vi "IT8800-Configure Range.vi"(6 "Numeric":dbl format="%#_13g", 8 "error in":errorcluster, 9 "Range":u16(ring) items=["MIN", "MAX", "DEFAULT"], 10 "Range Type":T2, 11 "IT8800 Setting In In":T1={"VISA Resource Name"="", "Baud Rate"=19200, "Stop Bits"=20, "Wait For Read(ms)"=0, "Interface Type"=enum."GPIB", "Limits"=[]} {"Stop Bits" items=["1.0"=10, "2.0"=20]; "Baud Rate" items=["2400"=2400, "4800"=4800, "9600"=9600, "19200"=19200]}) -> (0 "error out":errorcluster, 3 "IT8800 Setting In Out":T1={"VISA Resource Name"="", "Baud Rate"=19200, "Stop Bits"=20, "Wait For Read(ms)"=0, "Interface Type"=enum."GPIB", "Limits"=[]} {"Stop Bits" items=["1.0"=10, "2.0"=20]; "Baud Rate" items=["2400"=2400, "4800"=4800, "9600"=9600, "19200"=19200]})   [LabVIEW 2018]
doc: "Configures the current, voltage, power or conductance range."
uses:
  Data Def/IT8800-Operation Mode.ctl
  Data Def/IT8800-Setting.ctl
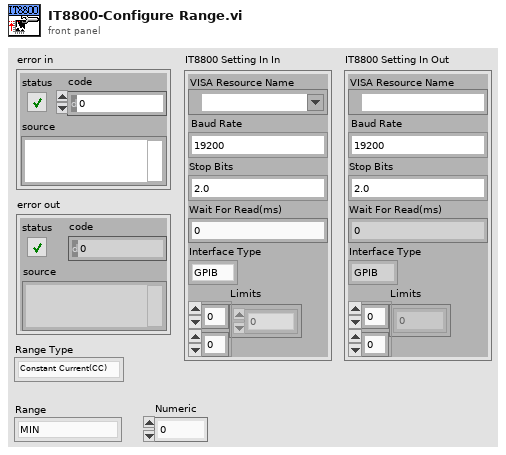
[diagram p1: front panel]
types:
  T1 = typedef "IT8800-Setting.ctl" = cluster{"VISA Resource Name":refnum<visa-resource-name>, "Baud Rate":u32, "Stop Bits":u16, "Wait For Read(ms)":u32, "Interface Type":enum16{"Unknow", "GPIB", "VXI", "GPIB-VXI", "Serial", "PXI", "TCPIP", "USB", "FireWire"}, "Limits":dbl[][]}
  T2 = typedef "IT8800-Operation Mode.ctl" = enum16{"Constant Current(CC)", "Constant Voltage(CV)", "Constant Power(CP)", "Constant Resistance(CR)"}
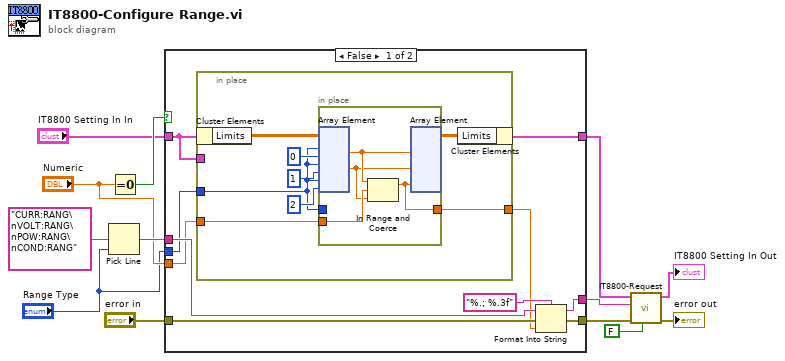
[diagram p0: block diagram]
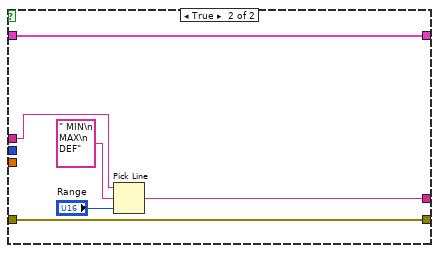
[diagram p2: hidden frame]
diagram:
  n1 = Pick Line(multi-line string="CURR:RANG\nVOLT:RANG\nPOW:RANG\nCOND:RANG", line index="Range Type") -> (output string=w12:string)  [unwired: 1 in]
  n2 = Equal To 0?(x="Numeric") -> (x = 0?=w7:bool)
  n3 = case shown="False" w7 {
    tunnel: w12 -> [w19 w41]
    tunnel: [w20 w38] -> w11
    tunnel: "Numeric" -> [w17 _]
    tunnel: "error in" -> [w22 w37]
    tunnel: [w21 w37] -> w4
    tunnel: "IT8800 Setting In In" -> [w15 w36]
    tunnel: "Range Type" -> [w18 _]
    tunnel: [w14 w36] -> w1
    frame False {
      n4 = in-place {
        in-place-border: w18 -> [w24]
        in-place-border: w17 -> [w31]
        in-place-border: [w30] -> w16
        in-place-border: w15 -> [_]
        n5 = in-place-cluster #1(w15) -> ("Limits"=w29:dbl[][])
        n6 = in-place {
          in-place-border: w24 -> [_]
          in-place-border: w31 -> [w35]
          in-place-border: [w32] -> w30
          n7 = in-place-array #2(w29, w24, 0, w24, 1, w24, 2) -> (w34:dbl, w33:dbl)  [unwired: 1 out]
          n8 = In Range and Coerce(upper limit=w34, x=w35, lower limit=w33) -> (coerced(x)=w32:dbl)  [unwired: 1 out]
          n9 = in-place-array #2(w34, w33, w32) -> (w28:dbl[][])  [unwired: 6 out]
        }
        n10 = in-place-cluster #1("Limits"=w28) -> (w14:T1)
      }
      n11 = Format Into String(format string="%.; %.3f", initial string=w19, error in=w22, w16) -> (resulting string=w20:string, error out=w21:errorcluster)
    }
    frame True {
      n12 = Pick Line(string ("")=w41, multi-line string=" MIN\n MAX\n DEF", line index="Range") -> (output string=w38:string)
    }
  }
  n13 = call "IT8800-Request.vi"("Response?"=FALSE, "error in"=w4, "Command"=w11, "IT8800 Setting In In"=w1) -> ("error out"=→"error out":errorcluster, "IT8800 Setting In Out"=→"IT8800 Setting In Out":T1)  [unwired: 5 in, 1 out]
